vi "Sequence - Power Up.vi"(8 "error in (no error)":errorcluster) -> (0 "error out":errorcluster)   [LabVIEW 2020]
uses:
  Library - Test Executive.llb/Test Executive.lvlib
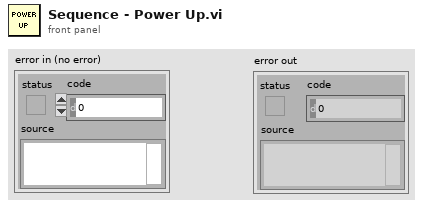
[diagram p1: front panel]
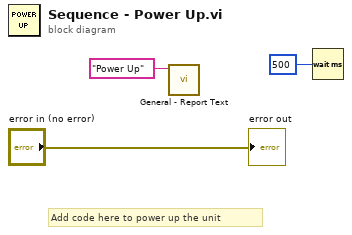
[diagram p0: block diagram]
diagram:
  # "Add code here to power up the unit"
  n1 = call "General - Report Text.vi"("Text In"="Power Up") -> ()  [unwired: 8 in, 3 out]
  n2 = Wait (ms)(milliseconds to wait=u32 500) -> ()  [unwired: 1 out]
  "error out" <- "error in (no error)"
